vi "PCO_SetLensFocus.vi"(8 "error in (no error)":errorcluster {"code" format="%x"}, 9 "dwflagsin":u32, 10 "lFocusPos":i32, 11 "hLens":u64) -> (0 "error out":errorcluster {"code" format="%x"}, 1 "lFocusPos out":i32, 2 "ErrorMessage":i32 format="%x", 3 "hLens out":u64, 5 "dwflagsout":u32)   [LabVIEW 2019, in "SDK.lvlib" / "LensControl.lvlib"]
doc: "<b>Description:</b>\nSets the focus of the lens control device to a new position. Value must be between 0...0x3FFF.\n\n<b>Supported camera type:</b>\npco.edge CLHS, pco.dimax cs\n\n<b>Descriptor dependency:</b>\nNone"
uses:
  LensControl.lvlib
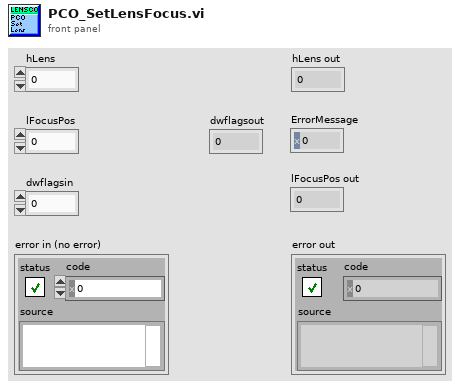
[diagram p1: front panel]
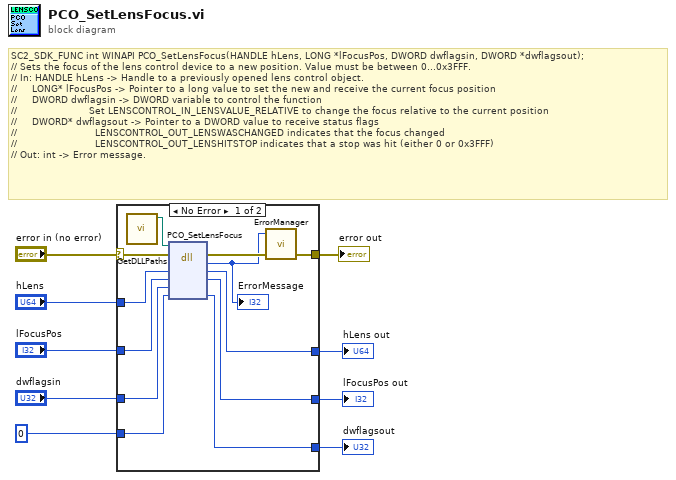
[diagram p0: block diagram]
diagram:
  # "SC2_SDK_FUNC int WINAPI PCO_SetLensFocus(HANDLE hLens, LONG *lFocusPos, DWORD dwflagsin, DWORD *dwflagsout);\n// Sets the focus of the lens control device to a new position. Value must be between 0...0x3FFF.\n// In: HANDLE hLens -> Handle to a previously opened lens control object.\n//     LONG* lFocusPos -> Pointer to a long value to set the new and receive the current focus position\n//     DWORD dwflagsin -> DWORD variable to control the function\n//                        Set LENSCONTROL_IN_LENSVALUE_RELATIVE to change the focus relative to the current position \n//     DWORD* dwflagsout -> Pointer to a DWORD value to receive status flags\n//                          LENSCONTROL_OUT_LENSWASCHANGED indicates that the focus changed\n//                          LENSCONTROL_OUT_LENSHITSTOP indicates that a stop was hit (either 0 or 0x3FFF)\n// Out: int -> Error message."
  n1 = case shown="No Error" "error in (no error)" {
    selector: "error in (no error)" -> [w14 w25]
    tunnel: "hLens" -> [w21 w24]
    tunnel: [w20 w24] -> w8
    tunnel: "lFocusPos" -> [w19 w23]
    tunnel: [w18 w23] -> w6
    tunnel: "dwflagsin" -> [w17 _]
    tunnel: u32 0 ("dwflagsout") -> [w16 w22]
    tunnel: [w15 w22] -> w3
    tunnel: [w13 w25] -> w2
    frame No Error {
      n2 = call "GetDLLPaths.vi"() -> ("SC2_Cam_Path"=w10:path)  [unwired: 9 in, 2 out]
      n3 = dll-call lib="?" fn="PCO_SetLensFocus"(path in=w10, error in=w14, "hLens"=w21, "lFocusPos"=w19, "dwflagsin"=w17, "dwflagsout"=w16) -> (error out=w12:errorcluster, "return type"=w11:i32, "hLens"=w20:u64, "lFocusPos"=w18:i32, "dwflagsout"=w15:u32)  [unwired: 2 in, 1 out]
      "ErrorMessage" <- w11
      n4 = call "ErrorManager.vi"("error in (no error)"=w12, "error code"=w11) -> ("error out"=w13:errorcluster)  [unwired: 3 in]
    }
    frame Error {
    }
  }
  "hLens out" <- w8
  "lFocusPos out" <- w6
  "dwflagsout" <- w3
  "error out" <- w2
